vi "Initialize E2E Configuration with Channels.vi"(8 "error in":errorcluster, 10 "Supported Channel Classifications (All)":T1[](array[typedef])=[enum."input data", enum."output data", enum."processing parameter", enum."processing result"]) -> (0 "error out":errorcluster, 2 "Random Channels Added":refnum<class "TBM channel.lvclass">[](array[class]), 3 "Initialized E2E configuration":refnum<class "E2E Tag Exchange configuration.lvclass">)   [LabVIEW 2015, in "E2E Tag Exchange tests.lvlib"]
uses:
  E2E Tag Exchange tests.lvlib
  module/configuration/E2E Tag Exchange configuration.lvclass
  <vilib>/NI/Tag Bus Module Framework/channel/TBM channel.lvclass
  <vilib>/NI/Tag Bus Module Framework/channel/channel classification.ctl
  <vilib>/NI/Configuration Framework/serializable configuration/NISE_CEF_serializable configuration.lvclass
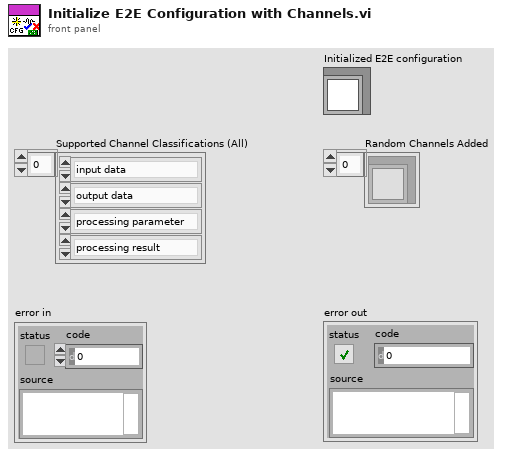
[diagram p1: front panel]
types:
  T1 = typedef "TBM channel.lvclass/channel classification.ctl" = enum16{"input data", "output data", "processing parameter", "processing result"}
  T2 = typedef "tag bus.lvlib/tag descriptor.lvclass/Data Type.ctl" = enum16{"Double", "Single", "I64", "I32", "I16", "I8", "U64", "U32", "U16", "U8", "Boolean", "String", "Array of Double", "Array of Single", "Array of I64", "Array of I32", "Array of I16", "Array of I8", "Array of U64", "Array of U32", "Array of U16", "Array of U8", "Array of Boolean", "Array of String"}
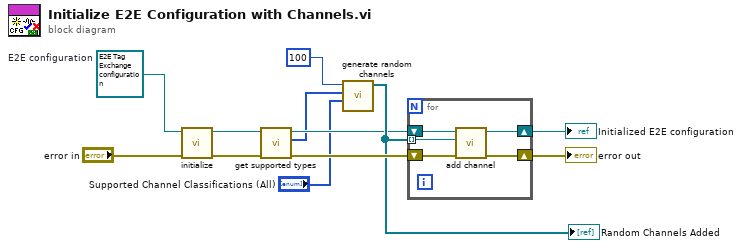
[diagram p0: block diagram]
diagram:
  w10 = refnum<class "E2E Tag Exchange configuration.lvclass"> refnum  # E2E configuration
  n1 = call <vilib>:"initialize.vi"("error in"="error in", "configuration in"=w10) -> ("error out"=w11:errorcluster, "configuration out"=w9:refnum<class "E2E Tag Exchange configuration.lvclass">)  [unwired: 7 in, 1 out]
  n2 = call-dynamic "get supported types.vi"("error in"=w11, "E2E Tag Exchange configuration in"=w9) -> ("error out"=w7:errorcluster, "supported types"=w3:T2[], "E2E Tag Exchange configuration out"=w5:refnum<class "E2E Tag Exchange configuration.lvclass">)  [unwired: 7 in]
  n3 = call "generate random channels.vi"("Supported Channel Classifications"="Supported Channel Classifications (All)", "supported types"=w3, "Number of Random Channels to Create"=100) -> ("Random Channels"=w6:refnum<class "TBM channel.lvclass">[])  [unwired: 8 in]
  "Random Channels Added" <- w6
  n4 = for {
    shift-right: [w16] -> w8
    shift-left: w5 -> [w17]
    tunnel: w6 -> [w15] mode=indexing
    shift-right: [w13] -> w12
    shift-left: w7 -> [w14]
    n5 = call "add channel.vi"("error in (no error)"=w14, "channel"=w15, "E2E configuration in"=w17) -> ("error out"=w13:errorcluster, "E2E configuration out"=w16:refnum<class "E2E Tag Exchange configuration.lvclass">)  [unwired: 7 in]
  }
  "error out" <- w12
  "Initialized E2E configuration" <- w8
